vi "Read Pressure (inHg).vi"(8 "error in (no error)":errorcluster, 11 "LPS Barometric Pressure Sensor in":refnum<class "LPS Barometric Pressure Sensor.lvclass">) -> (0 "error out":errorcluster, 2 "Pressure (inHg)":dbl, 3 "LPS Barometric Pressure Sensor out":refnum<class "LPS Barometric Pressure Sensor.lvclass">)   [LabVIEW 2020, in "LPS Barometric Pressure Sensor.lvclass"]
doc: "Read the pressure in scaled imperial units (inHg)."
uses:
  LPS Barometric Pressure Sensor.lvclass
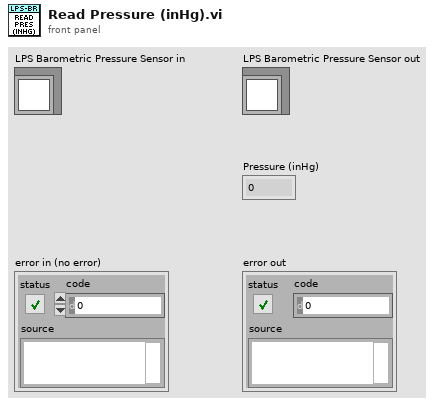
[diagram p1: front panel]
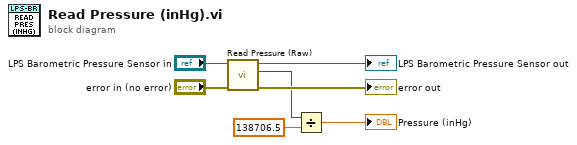
[diagram p0: block diagram]
diagram:
  n1 = call-dynamic "Read Pressure (Raw).vi"("error in (no error)"="error in (no error)", "LPS Barometer in"="LPS Barometric Pressure Sensor in") -> ("error out"=→"error out":errorcluster, "Raw Pressure"=w3:u32, "LPS Barometer out"=→"LPS Barometric Pressure Sensor out":refnum<class "LPS Barometric Pressure Sensor.lvclass">)  [unwired: 7 in]
  n2 = Divide(x=w3, y=138706.5) -> (x/y=→"Pressure (inHg)":dbl)
